vi "GlobalErrorCluster.vi"() -> ()   [LabVIEW 2013]
panel:
  in  "Medium Error Cluster":T1(array[cluster])
  in  "Error Cluster":T2(array[cluster])
  in  "Cluster Timestamps":dbl[](array[numeric])
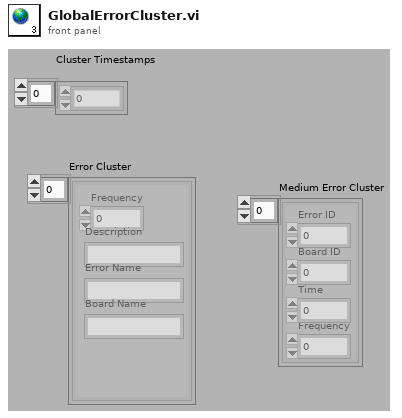
[diagram p1: front panel]
types:
  T1 = cluster{"Error ID":i32, "Board ID":i32, "Time":u32, "Frequency":i32}[]
  T2 = cluster{"Frequency":dbl, "Description":string, "Error Name":string, "Board Name":string}[]
diagram:
